vi "set async stop notifier.vi"(8 "error in":errorcluster {"code" format="Error %.0f"}, 10 "async stop notifier":refnum<notifier>, 11 "NATS Client in":refnum<class "NATS Client.lvclass">) -> (0 "error out":errorcluster {"code" format="Error %.0f"}, 3 "NATS Client out":refnum<class "NATS Client.lvclass">)   [LabVIEW 2024, in "NATS Client.lvlib" / "NATS Client.lvclass"]
uses:
  NATS Client.lvclass
  NATS Client.lvclass/NATS Client.ctl
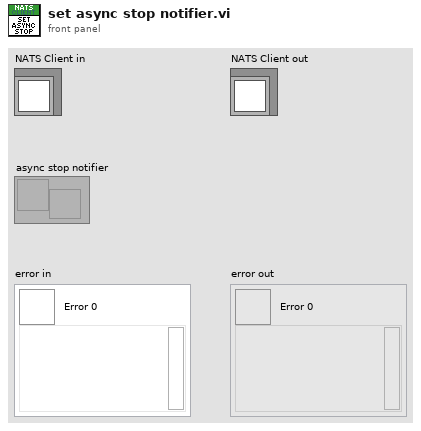
[diagram p1: front panel]
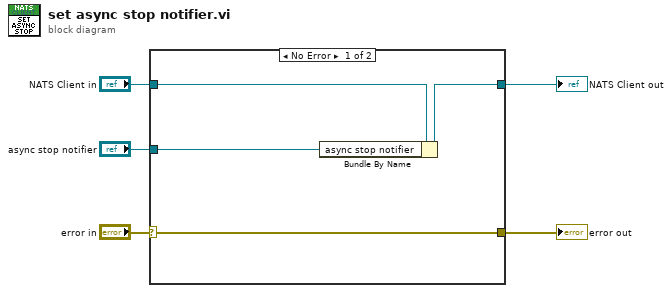
[diagram p0: block diagram]
diagram:
  n1 = case shown="No Error" "error in" {
    selector: "error in" -> [w9 w11]
    tunnel: [w9 w11] -> w4
    tunnel: [w7 w10] -> w2
    tunnel: "NATS Client in" -> [w8 w10]
    tunnel: "async stop notifier" -> [w6 _]
    frame No Error {
      n2 = Bundle By Name(cluster=w8, "async stop notifier"=w6) -> (w7:refnum<class "NATS Client.lvclass">)
    }
    frame Error {
    }
  }
  "error out" <- w4
  "NATS Client out" <- w2
